vi "FlatToRichcif_manager_QueryPluginResponse.vi"(5 "OutputClusterType":T1, 11 "InputCluster":T16) -> (3 "OutputCluster":T1)   [LabVIEW 2021, in "CIF_Manager_server.lvlib"]
uses:
  CIF_Manager_server.lvlib
  cif_manager_QueryPluginResponse_Flat.ctl
  cif_manager_PluginInfo_Flat.ctl
  cif_common_ShortVersion_Flat.ctl
  cif_management_common_PluginStatusData_Flat.ctl
  cif_management_common_PluginStatusData_PluginState.ctl
  cif_management_common_TimingStatistics_Flat.ctl
  cif_common_TimingStats_Flat.ctl
  cif_management_common_FifoStatistics_Flat.ctl
  cif_management_common_Error_Flat.ctl
  cif_management_common_MonitorDoubles_Flat.ctl
  cif_management_common_MonitorU64_Flat.ctl
  cif_management_common_MonitorI64_Flat.ctl
  cif_management_common_LoaderInfo_Flat.ctl
  cif_management_common_LoaderType.ctl
  cif_common_Status_Flat.ctl
  cif_manager_QueryPluginResponse.ctl
  cif_manager_PluginInfo.ctl
  cif_common_ShortVersion.ctl
  cif_management_common_PluginStatusData.ctl
  cif_management_common_TimingStatistics.ctl
  cif_common_TimingStats.ctl
  cif_management_common_FifoStatistics.ctl
  cif_management_common_Error.ctl
  cif_management_common_MonitorDoubles.ctl
  cif_management_common_MonitorU64.ctl
  cif_management_common_MonitorI64.ctl
  cif_management_common_LoaderInfo.ctl
  cif_common_Status.ctl
  FlatToRichcif_common_ShortVersion.vi
  FlatToRichcif_management_common_PluginStatusData.vi
  FlatToRichcif_management_common_LoaderInfo.vi
  FlatToRichcif_management_common_TimingStatistics.vi
  FlatToRichcif_management_common_FifoStatistics.vi
  FlatToRichcif_management_common_Error.vi
  FlatToRichcif_management_common_MonitorDoubles.vi
  FlatToRichcif_management_common_MonitorU64.vi
  FlatToRichcif_management_common_MonitorI64.vi
  FlatToRichcif_common_TimingStats.vi
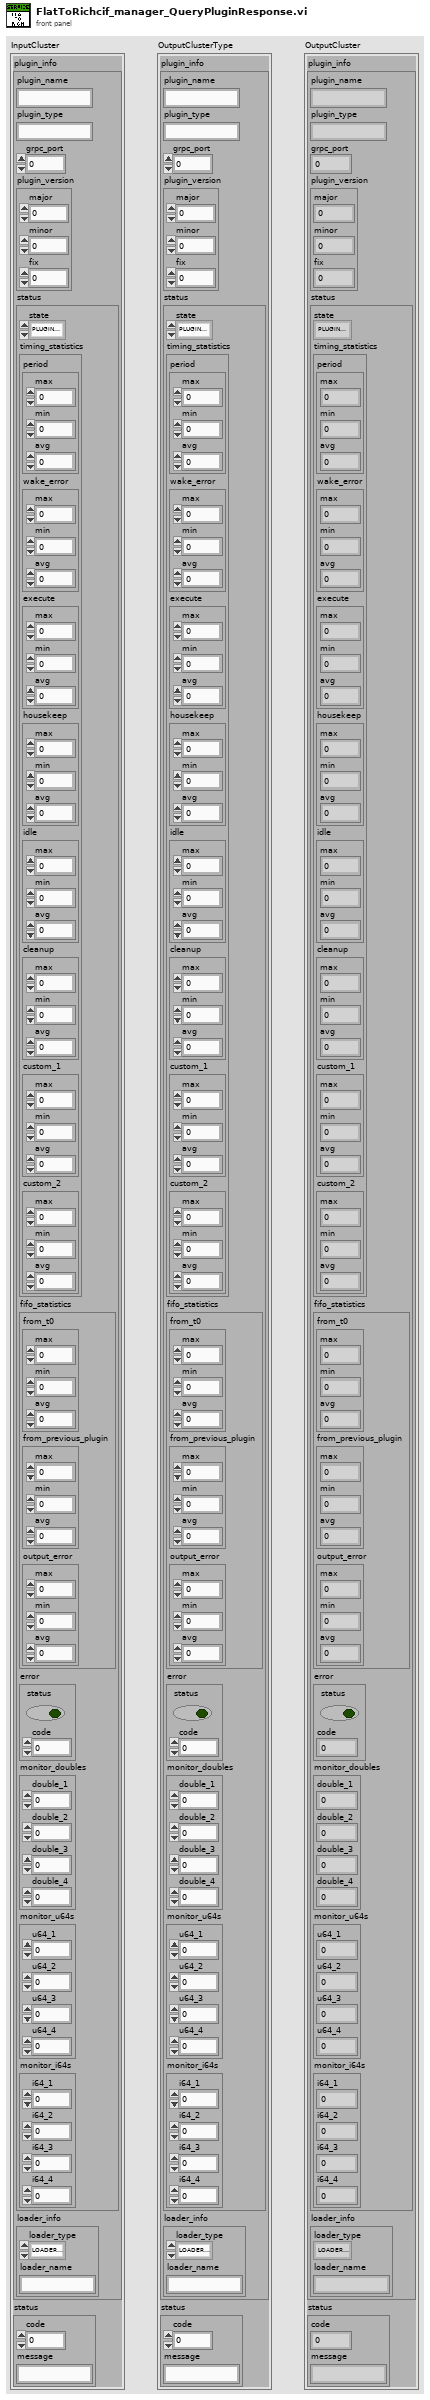
[diagram p1: front panel]
types:
  T1 = typedef "CIF_Manager_server.lvlib/cif_manager_QueryPluginResponse.ctl" = cluster{"plugin_info":T2, "status":T15}
  T2 = typedef "CIF_Manager_server.lvlib/cif_manager_PluginInfo.ctl" = cluster{"plugin_name":string, "plugin_type":string, "grpc_port":i32, "plugin_version":T3, "status":T4, "loader_info":T13}
  T3 = typedef "CIF_Manager_server.lvlib/cif_common_ShortVersion.ctl" = cluster{"major":u32, "minor":u32, "fix":u32}
  T4 = typedef "CIF_Manager_server.lvlib/cif_management_common_PluginStatusData.ctl" = cluster{"state":T5, "timing_statistics":T6, "fifo_statistics":T8, "error":T9, "monitor_doubles":T10, "monitor_u64s":T11, "monitor_i64s":T12}
  T5 = typedef "CIF_Manager_server.lvlib/cif_management_common_PluginStatusData_PluginState.ctl" = enum32{"PLUGINSTATE_UNKNOWN", "PLUGINSTATE_CREATING", "PLUGINSTATE_LISTENING", "PLUGINSTATE_RUNNING", "PLUGINSTATE_CLEANINGUP", "PLUGINSTATE_DESTROYING"}
  T6 = typedef "CIF_Manager_server.lvlib/cif_management_common_TimingStatistics.ctl" = cluster{"period":T7, "wake_error":T7, "execute":T7, "housekeep":T7, "idle":T7, "cleanup":T7, "custom_1":T7, "custom_2":T7}
  T7 = typedef "CIF_Manager_server.lvlib/cif_common_TimingStats.ctl" = cluster{"max":i64, "min":i64, "avg":dbl}
  T8 = typedef "CIF_Manager_server.lvlib/cif_management_common_FifoStatistics.ctl" = cluster{"from_t0":T7, "from_previous_plugin":T7, "output_error":T7}
  T9 = typedef "CIF_Manager_server.lvlib/cif_management_common_Error.ctl" = cluster{"status":bool, "code":i32}
  T10 = typedef "CIF_Manager_server.lvlib/cif_management_common_MonitorDoubles.ctl" = cluster{"double_1":dbl, "double_2":dbl, "double_3":dbl, "double_4":dbl}
  T11 = typedef "CIF_Manager_server.lvlib/cif_management_common_MonitorU64.ctl" = cluster{"u64_1":u64, "u64_2":u64, "u64_3":u64, "u64_4":u64}
  T12 = typedef "CIF_Manager_server.lvlib/cif_management_common_MonitorI64.ctl" = cluster{"i64_1":i64, "i64_2":i64, "i64_3":i64, "i64_4":i64}
  T13 = typedef "CIF_Manager_server.lvlib/cif_management_common_LoaderInfo.ctl" = cluster{"loader_type":T14, "loader_name":string}
  T14 = typedef "CIF_Manager_server.lvlib/cif_management_common_LoaderType.ctl" = enum32{"LOADERTYPE_UNKNOWN", "LOADERTYPE_LABVIEW"}
  T15 = typedef "CIF_Manager_server.lvlib/cif_common_Status.ctl" = cluster{"code":i32, "message":string}
  T16 = typedef "CIF_Manager_server.lvlib/cif_manager_QueryPluginResponse_Flat.ctl" = cluster{"plugin_info":T17, "status":T28}
  T17 = typedef "CIF_Manager_server.lvlib/cif_manager_PluginInfo_Flat.ctl" = cluster{"plugin_name":string, "plugin_type":string, "grpc_port":i32, "plugin_version":T18, "status":T19, "loader_info":T27}
  T18 = typedef "CIF_Manager_server.lvlib/cif_common_ShortVersion_Flat.ctl" = cluster{"major":u32, "minor":u32, "fix":u32}
  T19 = typedef "CIF_Manager_server.lvlib/cif_management_common_PluginStatusData_Flat.ctl" = cluster{"state":T5, "timing_statistics":T20, "fifo_statistics":T22, "error":T23, "monitor_doubles":T24, "monitor_u64s":T25, "monitor_i64s":T26}
  T20 = typedef "CIF_Manager_server.lvlib/cif_management_common_TimingStatistics_Flat.ctl" = cluster{"period":T21, "wake_error":T21, "execute":T21, "housekeep":T21, "idle":T21, "cleanup":T21, "custom_1":T21, "custom_2":T21}
  T21 = typedef "CIF_Manager_server.lvlib/cif_common_TimingStats_Flat.ctl" = cluster{"max":i64, "min":i64, "avg":dbl}
  T22 = typedef "CIF_Manager_server.lvlib/cif_management_common_FifoStatistics_Flat.ctl" = cluster{"from_t0":T21, "from_previous_plugin":T21, "output_error":T21}
  T23 = typedef "CIF_Manager_server.lvlib/cif_management_common_Error_Flat.ctl" = cluster{"status":bool, "code":i32}
  T24 = typedef "CIF_Manager_server.lvlib/cif_management_common_MonitorDoubles_Flat.ctl" = cluster{"double_1":dbl, "double_2":dbl, "double_3":dbl, "double_4":dbl}
  T25 = typedef "CIF_Manager_server.lvlib/cif_management_common_MonitorU64_Flat.ctl" = cluster{"u64_1":u64, "u64_2":u64, "u64_3":u64, "u64_4":u64}
  T26 = typedef "CIF_Manager_server.lvlib/cif_management_common_MonitorI64_Flat.ctl" = cluster{"i64_1":i64, "i64_2":i64, "i64_3":i64, "i64_4":i64}
  T27 = typedef "CIF_Manager_server.lvlib/cif_management_common_LoaderInfo_Flat.ctl" = cluster{"loader_type":T14, "loader_name":string}
  T28 = typedef "CIF_Manager_server.lvlib/cif_common_Status_Flat.ctl" = cluster{"code":i32, "message":string}
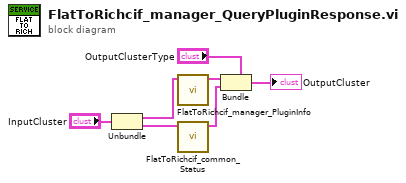
[diagram p0: block diagram]
diagram:
  n1 = Unbundle "Unbundle"("InputCluster") -> ("plugin_info"=w4:T17, "status"=w2:T28)
  n2 = call "FlatToRichcif_manager_PluginInfo.vi"("InputCluster"=w4) -> ("OutputCluster"=w3:T2)  [unwired: 10 in]
  n3 = call "FlatToRichcif_common_Status.vi"("InputCluster"=w2) -> ("OutputCluster"=w1:T15)  [unwired: 10 in]
  n4 = Bundle "Bundle"(cluster="OutputClusterType", "plugin_info"=w3, "status"=w1) -> (→"OutputCluster":T1)
